vi "New Action Sq1.vi"(9 "View":i32[](array[numeric]) caption="View (Team Index, -1: empty)", 10 "Team Index":i32, 11 "AndrewF in":refnum<class "AndrewF.lvclass">) -> (0 "Replicated":refnum<class "Square.lvclass">, 1 "Direction":T2, 2 "Action":T1, 3 "AndrewF out":refnum<class "AndrewF.lvclass">)   [LabVIEW 2016, in "AndrewF.lvclass"]
uses:
  AndrewF.lvclass
  C:/Users/crwec/Desktop/Workspace/SquareBattle/Square/Square.lvclass
  Square/Square.lvclass
  Type Defs/Direction Enum.ctl
  Type Defs/Action Enum.ctl
  AndrewF.lvclass/AndrewF.ctl
  Common/Common.lvlib
  Type Defs/SB Type Defs.lvlib
panel:
  # "NW\nN\nNE\nE\nSE\nS\nSW\nW"
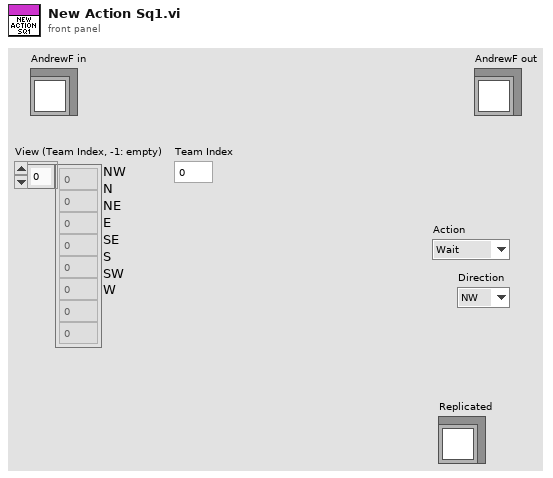
[diagram p1: front panel]
types:
  T1 = typedef "SB Type Defs.lvlib/Action Enum.ctl" = enum16{"Wait", "Move", "Attack", "Replicate"}
  T2 = typedef "SB Type Defs.lvlib/Direction Enum.ctl" = enum16{"NW", "N", "NE", "E", "SE", "S", "SW", "W"}
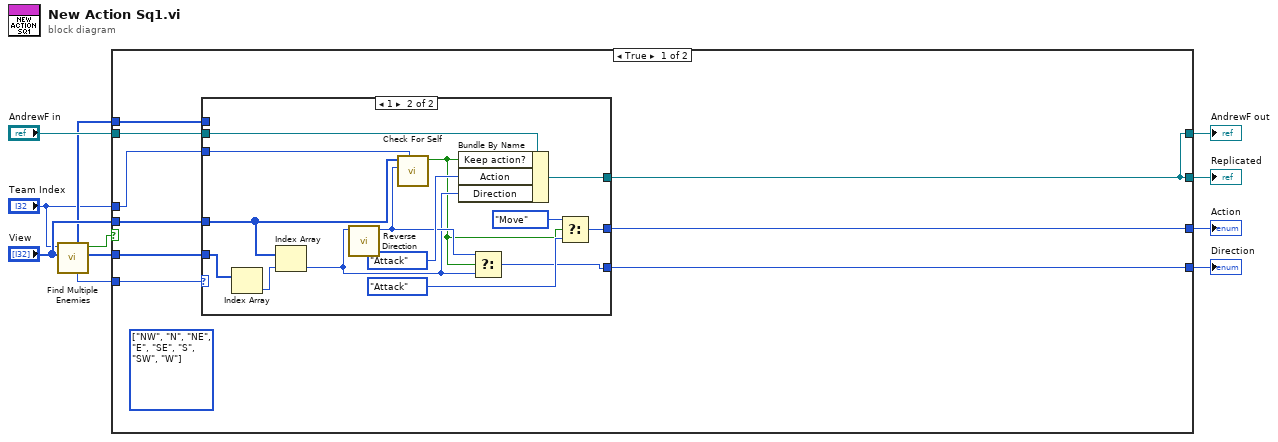
[diagram p0: block diagram]
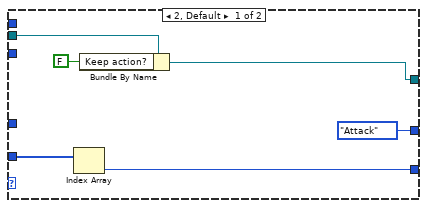
[diagram p2: hidden frame]
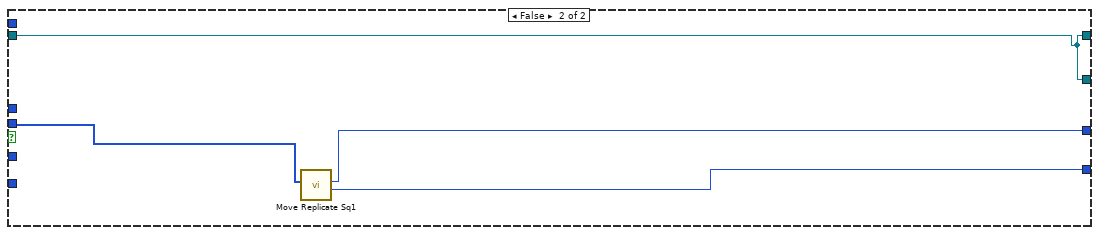
[diagram p3: hidden frame]
diagram:
  n1 = call "Find Multiple Enemies.vi"("View"="View", "Team Index"="Team Index") -> ("Direction"=w4:T2[], "Found Enemy?"=w2:bool, "How Many Enemies"=w3:i32, "Enemy"=w5:i32[])  [unwired: 6 in]
  n2 = case shown="True" w2 {
    tunnel: [w14 w41] -> w7
    tunnel: [w19 w42] -> w9
    tunnel: [w20 w43] -> w8
    tunnel: [w14 w41] -> w10
    tunnel: "AndrewF in" -> [w15 w41]
    tunnel: w3 -> [w18 _]
    tunnel: w4 -> [w17 _]
    tunnel: w5 -> [w16 _]
    tunnel: "View" -> [w13 w44]
    tunnel: "Team Index" -> [w12 _]
    frame True {
      (unwired) T2[] [enum."NW", enum."N", enum."NE", enum."E", enum."SE", enum."S", enum."SW", enum."W"] items=["NW", "N", "NE", "E", "SE", "S", "SW", "W"] ("Direction 2")
      n3 = case shown="1" w18 {
        tunnel: [Action_Enum."Attack" ("Action") w36] -> w20
        tunnel: [w23 w32] -> w19
        tunnel: w17 -> [w21 w29]
        tunnel: w16 -> [_ _]
        tunnel: w15 -> [w26 w40]
        tunnel: [w25 w39] -> w14
        tunnel: w13 -> [_ w30]
        tunnel: w12 -> [_ w27]
        frame 2, Default {
          n4 = Index Array(array=w21) -> (element=w23:T2)  [unwired: 1 in]
          n5 = Bundle By Name(cluster=w26, "Keep action?"=FALSE) -> (w25:refnum<class "AndrewF.lvclass">)
        }
        frame 1 {
          n6 = Index Array(array=w29) -> (element=w28:T2)  [unwired: 1 in]
          n7 = Index Array(array=w30, index=w28) -> (element=w33:i32)
          n8 = call "Reverse Direction.vi"("Direction in"=w33) -> ("Reverse Direction"=w34:i32)  [unwired: 10 in]
          n9 = call "Check For Self.vi"("Team index"=w27, "Direction"=w34, "Map"=w30) -> ("Clear?"=w31:bool)  [unwired: 8 in]
          n10 = Bundle By Name(cluster=w40, "Keep action?"=w31, "Action"=Action_Enum."Attack", "Direction"=w33) -> (w39:refnum<class "AndrewF.lvclass">)
          n11 = Select(t=w34, s=w31, f=w33) -> (s? t:f=w32:i32)
          n12 = Select(t=Action_Enum."Move" ("Action"), s=w31, f=Action_Enum."Attack") -> (s? t:f=w36:T1)
        }
      }
    }
    frame False {
      n13 = call "Move Replicate Sq1.vi"("View"=w44) -> ("Direction"=w42:T2, "Action"=w43:T1)  [unwired: 9 in]
    }
  }
  "AndrewF out" <- w10
  "Action" <- w8
  "Direction" <- w9
  "Replicated" <- w7
